vi "Write Analog Outputs.vi"(8 "error in (no error)":errorcluster, 9 "Device Number":string, 10 "Analog Outputs":dbl[](array[numeric]) min=0.0 max=10.0 step=0.0025, 11 "VISA resource name":refnum<visa-resource-name>) -> (0 "error out":errorcluster, 3 "VISA resource name out":refnum<visa-resource-name>)   [LabVIEW 2015, in "Zaber A Series.lvlib"]
doc: "Writes to the analog output pins on Zaber devices that have them. Input is an array of doubles that must have the same number of elements as there are analog output pins on the device - use the Get I/O Pin Counts VI to determine this.\n \nThis VI requires that the Initialize VI has been called with the same serial port."
uses:
  Zaber A Series.lvlib
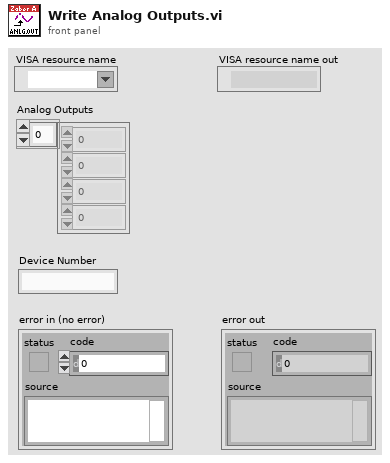
[diagram p1: front panel]
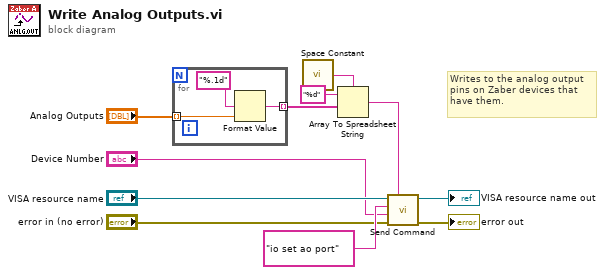
[diagram p0: block diagram]
diagram:
  # "Writes to the analog output\npins on Zaber devices that\nhave them."
  n1 = for {
    tunnel: [w14] -> w8 mode=indexing
    tunnel: "Analog Outputs" -> [w12] mode=indexing
    n2 = Format Value(format string="%.1d", value (0)=w12) -> (output string=w14:string)  [unwired: 1 in]
  }
  n3 = call <vilib>:"Space Constant.vi"() -> ("String"=w6:string)
  n4 = Array To Spreadsheet String(delimiter (Tab)=w6, array=w8, 3:"%d" ("format string")) -> (spreadsheet string=w5:string)
  n5 = call "Send Command.vi"("Data"=w5, "error in (no error)"="error in (no error)", "Device and Axis"="Device Number", "Command"="io set ao port" ("Complete Command List"), "VISA resource name"="VISA resource name") -> ("error out"=→"error out":errorcluster, "VISA resource name out"=→"VISA resource name out":refnum<visa-resource-name>)  [unwired: 1 in, 4 out]
